vi "Initialize_Globals.vi"(0 "ProFile Path":path, 1 "Energy":i16(slide)=100 min=0 max=100 step=1 scale=0.0..100.0, 2 "#Pulses":string="20", 3 "Step Size in mm":sgl=0.1, 4 "Offset Z-Axis":sgl, 5 "Y-Axis":sgl, 6 "Offset Y-Axis":sgl, 7 "X-Axis":sgl, 8 "Offset X-Axis":sgl) -> ()   [LabVIEW 2016]
uses:
  Global Constants.vi
  Global_Laser.vi
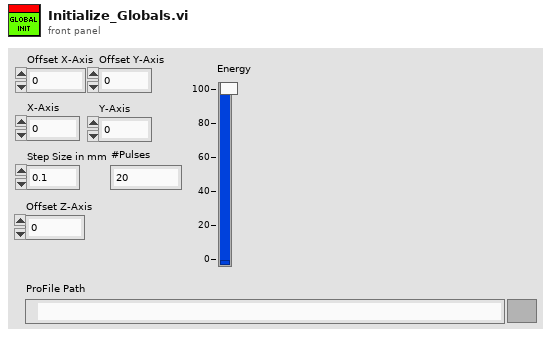
[diagram p1: front panel]
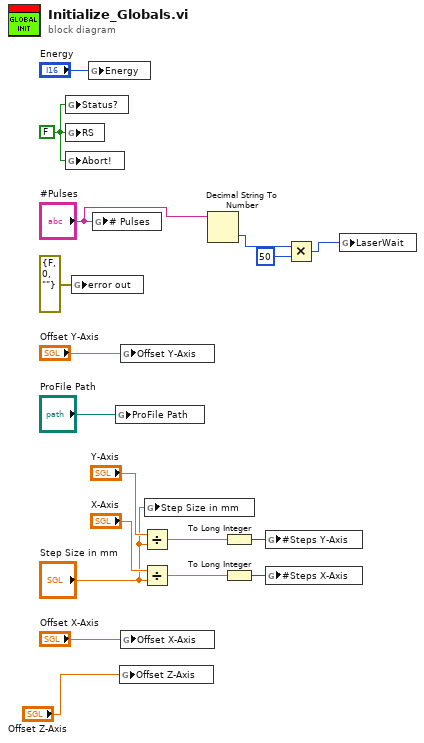
[diagram p0: block diagram]
diagram:
  w8 = FALSE
  n1 = global write "Global Constants.vi" "Status?"(w8) -> ()
  n2 = global write "Global Constants.vi" "RS"(w8) -> ()
  n3 = global write "Global Constants.vi" "Abort!"(w8) -> ()
  n4 = global write "Global Constants.vi" "error out"(errorcluster {"status"=FALSE, "code"=0, "source"=""} ("error")) -> ()
  n5 = global write "Global_Laser.vi" "Energy"("Energy") -> ()
  n6 = global write "Global_Laser.vi" "# Pulses"("#Pulses") -> ()
  n7 = global write "Global Constants.vi" "ProFile Path"("ProFile Path") -> ()
  n8 = global write "Global Constants.vi" "Offset Z-Axis"("Offset Z-Axis") -> ()
  n9 = global write "Global Constants.vi" "Offset Y-Axis"("Offset Y-Axis") -> ()
  n10 = global write "Global Constants.vi" "Offset X-Axis"("Offset X-Axis") -> ()
  n11 = Divide(x="Y-Axis", y="Step Size in mm") -> (x/y=w7:sgl)
  n12 = Divide(x="X-Axis", y="Step Size in mm") -> (x/y=w6:sgl)
  n13 = global write "Global Constants.vi" "Step Size in mm"("Step Size in mm") -> ()
  n14 = Decimal String To Number(string="#Pulses") -> (number=w3:i32)  [unwired: 2 in, 1 out]
  n15 = To Long Integer(number=w7) -> (32bit integer=w17:i32)
  n16 = To Long Integer(number=w6) -> (32bit integer=w18:i32)
  n17 = global write "Global Constants.vi" "#Steps Y-Axis"(w17) -> ()
  n18 = global write "Global Constants.vi" "#Steps X-Axis"(w18) -> ()
  n19 = Multiply(x=w3, y=50) -> (x*y=w1:i32)
  n20 = global write "Global_Laser.vi" "LaserWait"(w1) -> ()
